vi "MenuStrip Example.vi"() -> ()   [LabVIEW 2016]
doc: "Demonstrates the Menu Strip type. Run the VI to see the menu appear in the MenuStrip .NET control. Notice the \"File-> Default\"menu item that contains an icon as well as the \"File->Exit\" menu item contains a shortcut.\n\nClick summarys show up in the history array. Click the \"Add Item\" to add a dummy item to the MenuStrip's menu."
uses:
  System.Windows.Forms
  <userlib>/_MGI/Menu Building/SelectionType/RadioSelection/MGI_RadioSelection.lvclass
  C:/Program Files (x86)/National Instruments/LabVIEW 2016/user.lib/_MGI/Menu Building/SelectionType/MGI_SelectionType.lvclass
  <userlib>/_MGI/Menu Building/SelectionType/CheckmarkSelection/MGI_CheckmarkSelection.lvclass
  <userlib>/_MGI/Menu Building/MenuItem/MenuStripItem/MGI_MenuStripItem.lvclass
  C:/Program Files (x86)/National Instruments/LabVIEW 2016/user.lib/_MGI/Menu Building/MenuItem/MGI_MenuItem.lvclass
  <userlib>/_MGI/Menu Building/MenuItem/MenuSeparatorItem/MGI_MenuSeparatorItem.lvclass
  <userlib>/_MGI/Menu Building/MenuTypes/MenuStrip/MGI_MenuStrip.lvclass
  C:/Program Files (x86)/National Instruments/LabVIEW 2016/user.lib/_MGI/Menu Building/MenuTypes/MGI_Menu.lvclass
  <userlib>/_MGI/Menu Building/MenuTypes/MenuStrip/MenuStrip.vi
  <userlib>/_MGI/Menu Building/MenuItem/MenuItem.vi
  <userlib>/_MGI/Menu Building/SelectionType/RadioSelection/RadioSelection.vi
  <userlib>/_MGI/Menu Building/MenuItem/Write Click By Default.vi
  <userlib>/_MGI/Menu Building/MenuItem/Write Sub-Menus.vi
  <userlib>/_MGI/Menu Building/MenuItem/MenuStripItem/MenuStripItem.vi
  <userlib>/_MGI/Menu Building/MenuItem/MenuSeparatorItem/MenuSeparatorItem.vi
  <userlib>/_MGI/Menu Building/SelectionType/CheckmarkSelection/CheckmarkSelection.vi
  <userlib>/_MGI/Menu Building/MenuItem/Read Sub-Menus.vi
  <userlib>/_MGI/Menu Building/MenuTypes/Read Menu Items.vi
  <userlib>/_MGI/Menu Building/MenuItem/MGI_MenuItem.lvclass
  <userlib>/_MGI/Menu Building/SelectionType/MGI_SelectionType.lvclass
  <userlib>/_MGI/Menu Building/MenuTypes/MGI_Menu.lvclass
  <userlib>/_MGI/Menu Building/MenuItemStatusChange/MGI_MenuItemStatusChange.lvclass
panel:
  in  "Add Item":bool
  out "History":T1(array[cluster])
  in  "MenuStrip":refnum<k24>(container)
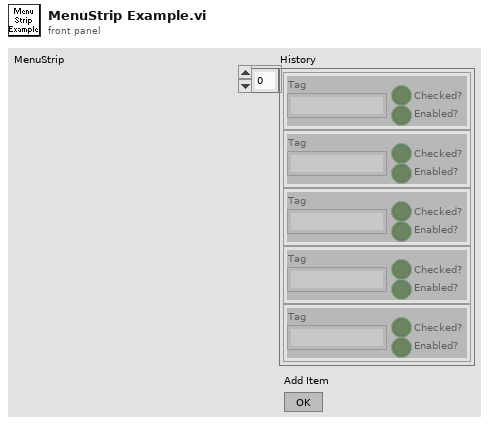
[diagram p1: front panel]
types:
  T1 = cluster{"Tag":string, "Checked?":bool, "Enabled?":bool}[]
  T2 = cluster{"Tag":string, "Checked?":bool, "Enabled?":bool}
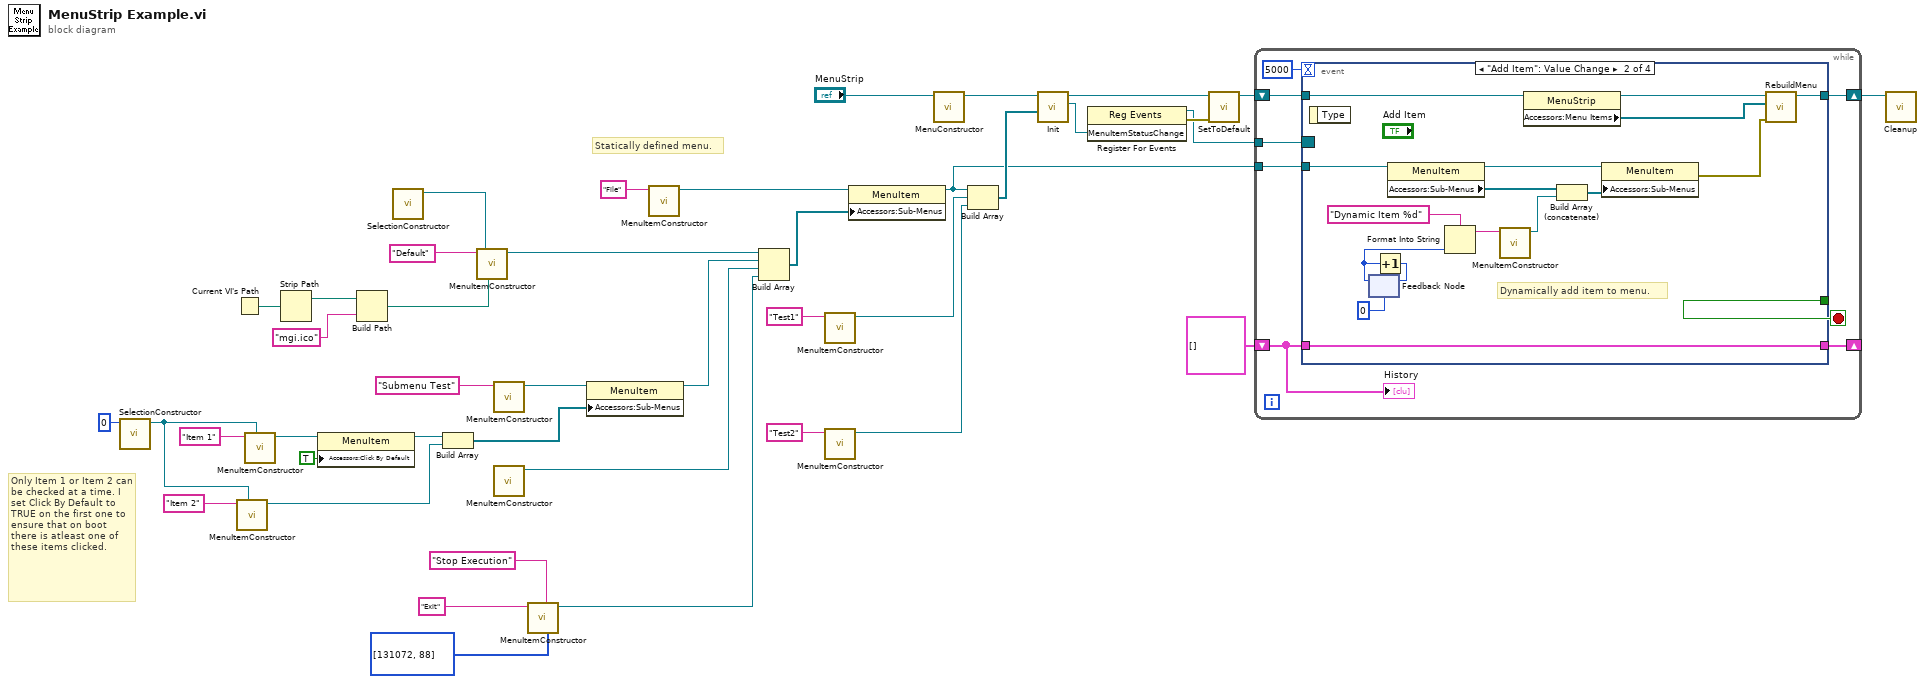
[diagram p0: block diagram]
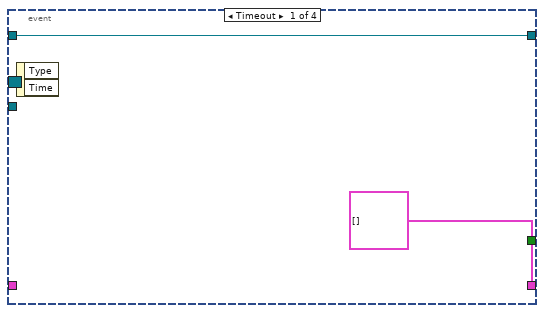
[diagram p2: hidden frame]
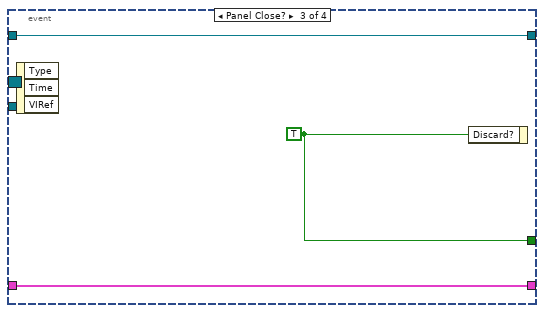
[diagram p3: hidden frame]
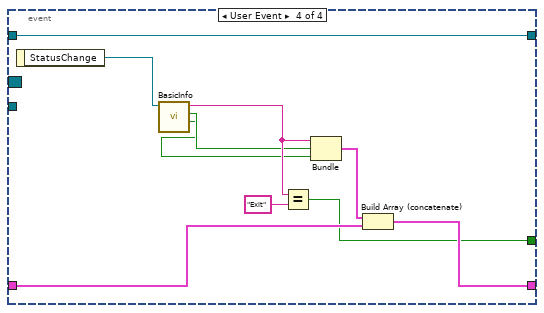
[diagram p4: hidden frame]
diagram:
  w12 = i32[] [131072, 88] items=["None"=0, "LButton"=1, "RButton"=2, "Cancel"=3, "MButton"=4, "XButton1"=5, "XButton2"=6, "Back"=8, "Tab"=9, "LineFeed"=10, "Clear"=12, "Enter, Return"=13, "ShiftKey"=16, "ControlKey"=17, "Menu"=18, "Pause"=19, "CapsLock, Capital"=20, "HangulMode, HanguelMode, KanaMode"=21, "JunjaMode"=23, "FinalMode"=24, "KanjiMode, HanjaMode"=25, "Escape"=27, "IMEConvert"=28, "IMENonconvert"=29, "IMEAccept, IMEAceept"=30, "IMEModeChange"=31, "Space"=32, "Prior, PageUp"=33, "PageDown, Next"=34, "End"=35, "Home"=36, "Left"=37, "Up"=38, "Right"=39, "Down"=40, "Select"=41, "Print"=42, "Execute"=43, "Snapshot, PrintScreen"=44, "Insert"=45, "Delete"=46, "Help"=47, "D0"=48, "D1"=49, "D2"=50, "D3"=51, "D4"=52, "D5"=53, "D6"=54, "D7"=55, "D8"=56, "D9"=57, "A"=65, "B"=66, "C"=67, "D"=68, "E"=69, "F"=70, "G"=71, "H"=72, "I"=73, "J"=74, "K"=75, "L"=76, "M"=77, "N"=78, "O"=79, "P"=80, "Q"=81, "R"=82, "S"=83, "T"=84, "U"=85, "V"=86, "W"=87, "X"=88, "Y"=89, "Z"=90, "LWin"=91, "RWin"=92, "Apps"=93, "Sleep"=95, "NumPad0"=96, "NumPad1"=97, "NumPad2"=98, "NumPad3"=99, "NumPad4"=100, "NumPad5"=101, "NumPad6"=102, "NumPad7"=103, "NumPad8"=104, "NumPad9"=105, "Multiply"=106, "Add"=107, "Separator"=108, "Subtract"=109, "Decimal"=110, "Divide"=111, "F1"=112, "F2"=113, "F3"=114, "F4"=115, "F5"=116, "F6"=117, "F7"=118, "F8"=119, "F9"=120, "F10"=121, "F11"=122, "F12"=123, "F13"=124, "F14"=125, "F15"=126, "F16"=127, "F17"=128, "F18"=129, "F19"=130, "F20"=131, "F21"=132, "F22"=133, "F23"=134, "F24"=135, "NumLock"=144, "Scroll"=145, "LShiftKey"=160, "RShiftKey"=161, "LControlKey"=162, "RControlKey"=163, "LMenu"=164, "RMenu"=165, "BrowserBack"=166, "BrowserForward"=167, "BrowserRefresh"=168, "BrowserStop"=169, "BrowserSearch"=170, "BrowserFavorites"=171, "BrowserHome"=172, "VolumeMute"=173, "VolumeDown"=174, "VolumeUp"=175, "MediaNextTrack"=176, "MediaPreviousTrack"=177, "MediaStop"=178, "MediaPlayPause"=179, "LaunchMail"=180, "SelectMedia"=181, "LaunchApplication1"=182, "LaunchApplication2"=183, "OemSemicolon, Oem1"=186, "Oemplus"=187, "Oemcomma"=188, "OemMinus"=189, "OemPeriod"=190, "Oem2, OemQuestion"=191, "Oem3, Oemtilde"=192, "Oem4, OemOpenBrackets"=219, "OemPipe, Oem5"=220, "OemCloseBrackets, Oem6"=221, "OemQuotes, Oem7"=222, "Oem8"=223, "Oem102, OemBackslash"=226, "ProcessKey"=229, "Packet"=231, "Attn"=246, "Crsel"=247, "Exsel"=248, "EraseEof"=249, "Play"=250, "Zoom"=251, "NoName"=252, "Pa1"=253, "OemClear"=254, "KeyCode"=65535, "Shift"=65536, "Control"=131072, "Alt"=262144, "Modifiers"=-65536] ("Shortcut Keys")
  # "Only Item 1 or Item 2 can be checked at a time. I set Click By Default to TRUE on the first one to ensure that on boot there is atleast one of these items clicked."
  # "Statically defined menu."
  n1 = call-poly <userlib>:"SelectionConstructor.vi"("Group"=u8 0) -> ("RadioSelection out"=w22:refnum<class "MGI_RadioSelection.lvclass">)  [unwired: 9 in, 1 out]
  n2 = Current VI's Path() -> (path=w6:path)
  n3 = call-poly <userlib>:"MenuItemConstructor.vi"("Selection Type"=w22, "Text"="Item 2") -> ("MenuItem"=w24:refnum<data-value>)  [unwired: 8 in, 1 out]
  n4 = call-poly <userlib>:"MenuItemConstructor.vi"("Selection Type"=w22, "Text"="Item 1") -> ("MenuItem"=w27:refnum<data-value>)  [unwired: 8 in, 1 out]
  n5 = Strip Path(path=w6) -> (stripped path=w5:path)  [unwired: 1 out]
  n6 = property class="MenuItem"(reference=w27, "Accessors:Click By Default"=TRUE ("Click By Default")) -> (reference out=w21:refnum<data-value>)  [unwired: 1 in, 1 out]
  n7 = Build Path(base path=w5, name or relative path="mgi.ico") -> (appended path=w3:path)
  n8 = call-poly <userlib>:"SelectionConstructor.vi"() -> ("CheckmarkSelection out"=w11:refnum<class "MGI_CheckmarkSelection.lvclass">)  [unwired: 10 in, 1 out]
  n9 = Build Array(w21, w24) -> (w35:refnum<data-value>[])
  n10 = call-poly <userlib>:"MenuItemConstructor.vi"("Icon"=w3, "SelectionType"=w11, "Text"="Default") -> ("MenuStripItem"=w9:refnum<data-value>)  [unwired: 7 in, 1 out]
  n11 = call-poly <userlib>:"MenuItemConstructor.vi"("Text"="Submenu Test") -> ("MenuItem"=w29:refnum<data-value>)  [unwired: 9 in, 1 out]
  n12 = call-poly <userlib>:"MenuItemConstructor.vi"() -> ("MenuSeparatorItem"=w28:refnum<data-value>)  [unwired: 10 in, 1 out]
  n13 = call-poly <userlib>:"MenuItemConstructor.vi"("Shortcut Keys"=w12, "ToolTip"="Stop Execution", "Text"="Exit") -> ("MenuStripItem"=w15:refnum<data-value>)  [unwired: 7 in, 1 out]
  n14 = property class="MenuItem"(reference=w29, "Accessors:Sub-Menus"=w35) -> (reference out=w34:refnum<data-value>)  [unwired: 1 in, 1 out]
  n15 = call-poly <userlib>:"MenuItemConstructor.vi"("Text"="File") -> ("MenuItem"=w32:refnum<data-value>)  [unwired: 9 in, 1 out]
  n16 = Build Array(w9, w34, w28, w15) -> (w33:refnum<data-value>[])
  n17 = call-poly <userlib>:"MenuItemConstructor.vi"("Text"="Test1") -> ("MenuItem"=w18:refnum<data-value>)  [unwired: 9 in, 1 out]
  n18 = call-poly <userlib>:"MenuItemConstructor.vi"("Text"="Test2") -> ("MenuItem"=w16:refnum<data-value>)  [unwired: 9 in, 1 out]
  n19 = property class="MenuItem"(reference=w32, "Accessors:Sub-Menus"=w33) -> (reference out=w1:refnum<data-value>)  [unwired: 1 in, 1 out]
  n20 = call-poly <userlib>:"MenuConstructor.vi"("MenuStrip"="MenuStrip") -> ("MenuStrip out"=w7:refnum<class "MGI_MenuStrip.lvclass">)  [unwired: 9 in, 1 out]
  n21 = Build Array(w1, w18, w16) -> (w37:refnum<data-value>[])
  n22 = call-dynamic "Init.vi"("Menu Items"=w37, "Menu in"=w7) -> ("MenuItemStatusChange"=w42:refnum<user-event>, "Menu out"=w41:refnum<class "MGI_MenuStrip.lvclass">)  [unwired: 7 in, 1 out]
  n23 = register-events(w42) -> (reference out=w36:refnum<event-registration>, error out=w40:errorcluster)  [unwired: 2 in]
  n24 = call-dynamic "SetToDefault.vi"("error in (no error)"=w40, "Menu in"=w41) -> ("Menu out"=w39:refnum<class "MGI_MenuStrip.lvclass">)  [unwired: 8 in, 1 out]
  n25 = while {
    shift-right: [w48] -> w38
    shift-left: w39 -> [w50]
    tunnel: w36 -> [w47]
    shift-right: [w46] -> _
    shift-left: T1 [] -> [w45]
    tunnel: w1 -> [w43]
    stop <- w49 stop-if-true
    n26 = event shown="[1] \"Add Item\": Value Change" {
      selector: w47 -> [_ _ _ _]
      dyn-events: _ -> [_ _ _ _]
      timeout: 5000 -> [_ _ _ _]
      tunnel: w50 -> [w52 w61 w70 w81]
      tunnel: [_ _ w71 w77] -> w49
      tunnel: [w52 w60 w70 w81] -> w48
      tunnel: w45 -> [_ w68 w69 w79]
      tunnel: [T1 [] w68 w69 w80] -> w46
      tunnel: w43 -> [_ w58 _ _]
      event Timeout {
        n27 = event-data() -> ()  [unwired: 1 in, 2 out]
      }
      event "Add Item": Value Change {
        # "Dynamically add item to menu."
        n28 = event-data() -> ()  [unwired: 1 in, 1 out]
        n29 = feedback #1(0) -> (w64:i32)
        n30 = Increment(x=w64) -> (x+1=w63:i32)
        n31 = feedback-in #1(w63) -> ()
        n32 = property class="MenuItem"(reference=w58) -> (reference out=w55:refnum<data-value>, "Accessors:Sub-Menus"=w57:refnum<data-value>[])  [unwired: 1 in, 1 out]
        n33 = Format Into String(format string="Dynamic Item %d" ("Text"), w64) -> (resulting string=w62:string)  [unwired: 2 in, 1 out]
        n34 = call-poly <userlib>:"MenuItemConstructor.vi"("Text"=w62) -> ("MenuItem"=w56:refnum<data-value>)  [unwired: 9 in, 1 out]
        n35 = property class="MenuStrip"(reference=w61) -> (reference out=w67:refnum<class "MGI_MenuStrip.lvclass">, "Accessors:Menu Items"=w59:refnum<data-value>[])  [unwired: 1 in, 1 out]
        n36 = Build Array (concatenate)(w57, w56) -> (w54:refnum<data-value>[])
        n37 = property class="MenuItem"(reference=w55, "Accessors:Sub-Menus"=w54) -> (error out=w53:errorcluster)  [unwired: 1 in, 1 out]
        n38 = call <userlib>:"RebuildMenu.vi"("error in (no error)"=w53, "New Menu Items"=w59, "Menu in"=w67) -> ("Menu out"=w60:refnum<class "MGI_MenuStrip.lvclass">)  [unwired: 7 in, 1 out]
      }
      event Panel Close? {
        w71 = TRUE ("Discard?")
        n39 = event-data() -> ()  [unwired: 1 in, 3 out]
        n40 = event-data("Discard?"=w71) -> ()  [unwired: 1 in, 1 out]
      }
      event User Event {
        n41 = event-data() -> ("StatusChange"=w76:refnum<class "MGI_MenuItemStatusChange.lvclass">)  [unwired: 1 in]
        n42 = call <userlib>:"BasicInfo.vi"("MGI_MenuItemStatusChange in"=w76) -> ("Enabled?"=w73:bool, "Checked?"=w74:bool, "Tag"=w75:string)  [unwired: 7 in, 1 out]
        n43 = Equal?(x=w75, y="Exit") -> (x = y?=w77:bool)
        n44 = Bundle("Tag"=w75, "Checked?"=w74, "Enabled?"=w73) -> (w72:T2)  [unwired: 1 in]
        n45 = Build Array (concatenate)(w72, w79) -> (w80:T1)
      }
    }
    "History" <- w45
  }
  n46 = call-dynamic "Cleanup.vi"("MenuStrip in"=w38) -> ()  [unwired: 10 in, 1 out]
